vi "arduinoSetPositionServo.vi"(0 "speed":u8 max=63 step=1, 1 "servo position":u16(knob)=260 max=2500 step=1 scale=260.0..1150.0, 2 "channel":u8 max=15 step=1) -> ()   [LabVIEW 2012]
uses:
  GlobalArduino.vi
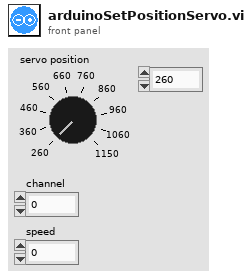
[diagram p1: front panel]
types:
  T1 = typedef "Semaphore RefNum" = refnum<k1>
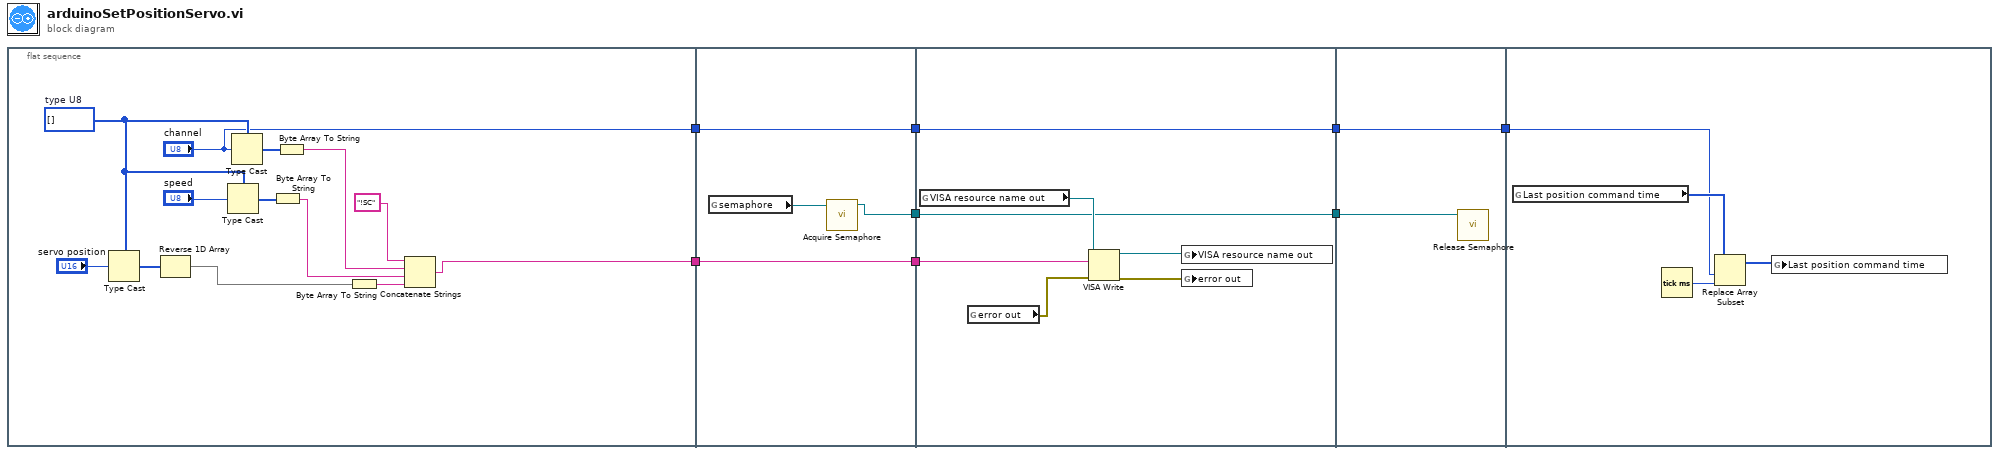
[diagram p0: block diagram]
diagram:
  n1 = flat-sequence {
    tunnel: ["channel"] -> w8
    tunnel: [w9] -> w6
    tunnel: w8 -> [w25]
    tunnel: [w25] -> w7
    tunnel: w6 -> [w24]
    tunnel: [w24] -> w5
    tunnel: [w22] -> w2
    tunnel: w7 -> [w32]
    tunnel: [w32] -> w4
    tunnel: w5 -> [w27]
    tunnel: w2 -> [w26]
    tunnel: [w26] -> w1
    tunnel: w4 -> [w34]
    tunnel: [w34] -> w3
    tunnel: w1 -> [w33]
    tunnel: w3 -> [w36]
    frame #0 {
      w15 = u8[] []  # type U8
      n2 = Type Cast(type=w15, x="servo position") -> (*(type *) &x=w18:u8[])
      n3 = Reverse 1D Array(array=w18) -> (reversed array=w11:u8[])
      n4 = Type Cast(type=w15, x="speed") -> (*(type *) &x=w14:u8[])
      n5 = Type Cast(type=w15, x="channel") -> (*(type *) &x=w16:u8[])
      n6 = Byte Array To String(unsigned byte array=w14) -> (string=w13:string)
      n7 = Byte Array To String(unsigned byte array=w16) -> (string=w17:string)
      n8 = Byte Array To String(unsigned byte array=w11) -> (string=w19:string)
      n9 = Concatenate Strings("!SC" ("string"), w17, w13, w19) -> (w9:string)
    }
    frame #1 {
      n10 = global read "GlobalArduino.vi" "semaphore"() -> (w23:T1)
      n11 = call <vilib>:"Acquire Semaphore.vi"("semaphore"=w23) -> ("semaphore out"=w22:T1)  [unwired: 4 in, 2 out]
    }
    frame #2 {
      n12 = global read "GlobalArduino.vi" "VISA resource name out"() -> (w28:refnum<visa-resource-name>)
      n13 = global read "GlobalArduino.vi" "error out"() -> (w30:errorcluster)
      n14 = VISA Write(VISA resource name=w28, write buffer=w27, error in (no error)=w30) -> (VISA resource name out=w29:refnum<visa-resource-name>, error out=w31:errorcluster)  [unwired: 1 out]
      n15 = global write "GlobalArduino.vi" "VISA resource name out"(w29) -> ()
      n16 = global write "GlobalArduino.vi" "error out"(w31) -> ()
    }
    frame #3 {
      n17 = call <vilib>:"Release Semaphore.vi"("semaphore"=w33) -> ()  [unwired: 5 in, 2 out]
    }
    frame #4 {
      n18 = global read "GlobalArduino.vi" "Last position command time"() -> (w37:u64[])
      n19 = Tick Count (ms)() -> (millisecond timer value=w35:u32)
      n20 = Replace Array Subset(array=w37, new element=w35, index=w36) -> (w38:u64[])
      n21 = global write "GlobalArduino.vi" "Last position command time"(w38) -> ()
    }
  }
